vi "Error Handlers (Single).vi"(8 "error in (no error)":errorcluster, 9 "error code":i32, 10 "condition failed?":bool) -> (0 "error out":errorcluster)   [LabVIEW 2017, in "NI_AAL_Filter.lvlib"]
uses:
  <vilib>/Analysis/NI_AAL_Filter.lvlib
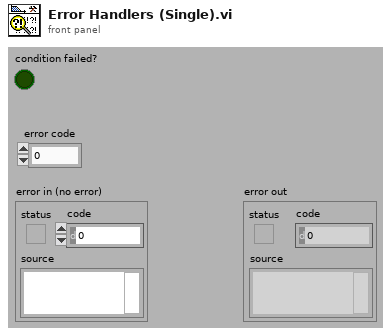
[diagram p1: front panel]
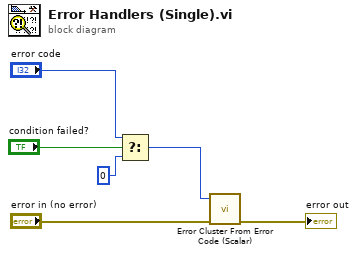
[diagram p0: block diagram]
diagram:
  n1 = Select(t="error code", s="condition failed?", f=0) -> (s? t:f=w1:i32)
  n2 = call <vilib>:"Error Cluster From Error Code (Scalar).vi"("error in (no error)"="error in (no error)", "error code (0)"=w1) -> ("error out"=→"error out":errorcluster)  [unwired: 9 in]
